vi "SENS_FREQ_STAR.vi"(0 "VISA IN":refnum<visa-resource-name>, 1 "Frq. Start":dbl, 5 "error in":errorcluster, 7 "Channel":i32=1) -> (14 "VISA Out":refnum<visa-resource-name>, 19 "error out":errorcluster)   [LabVIEW 2018, in "PNA-X.lvlib"]
doc: "SENSe<cnum>:FREQuency:STARt <num> \n1745\n\n(Read-Write) Sets the start frequency of the analyzer. \nParameters \n<cnum> Any existing channel number. If unspecified, value is set to 1 \n<num> Start frequency. Choose any number between the MIN and MAX frequency \nlimits of the analyzer. Units are Hz \nIf FREQ:START is set greater than FREQ:STOP, then STOP is set equal to \nSTART. \nSee Note \nExamples SENS:FREQ:STAR 1000000 \nsense2:frequency:start MIN \nQuery Syntax SENSe<cnum>:FREQuency:STARt? \nIf Sweep type is segment, this query returns the start frequency of the first \nsegment. \nReturn Type Numeric \nDefault Minimum frequency of the analyzer"
uses:
  PNA-X.lvlib
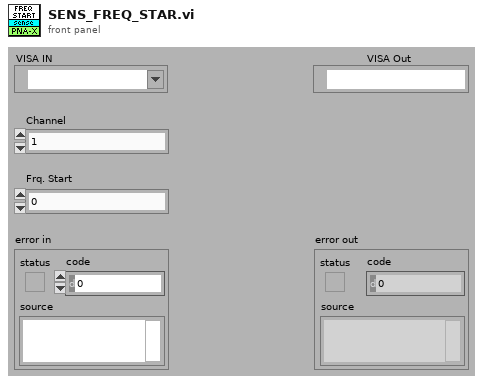
[diagram p1: front panel]
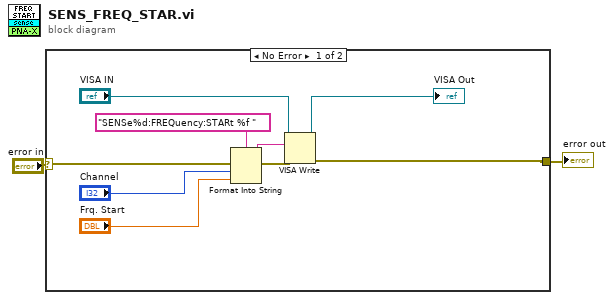
[diagram p0: block diagram]
diagram:
  n1 = case shown="No Error" "error in" {
    selector: "error in" -> [w11 w12]
    tunnel: [w6 w12] -> w1
    frame No Error {
      n2 = Format Into String(format string="SENSe%d:FREQuency:STARt %f " ("Cmdline"), error in=w11, "Channel", "Frq. Start") -> (resulting string=w9:string, error out=w10:errorcluster)  [unwired: 1 in]
      n3 = VISA Write(VISA resource name="VISA IN", write buffer=w9, error in (no error)=w10) -> (VISA resource name out=→"VISA Out":refnum<visa-resource-name>, error out=w6:errorcluster)  [unwired: 1 out]
    }
    frame Error {
    }
  }
  "error out" <- w1
